vi "Get Send Type.vi"(11 "Message Scripter in":refnum<class "Message Scripter.lvclass">) -> (2 "Send Type":enum16{"Concrete", "Abstract"}(ring))   [LabVIEW 2020, in "Message Maker.lvlib" / "Message Scripter.lvclass"]
uses:
  Message Scripter.lvclass
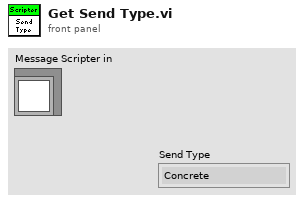
[diagram p1: front panel]
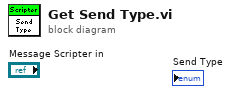
[diagram p0: block diagram]
diagram:
